vi "Set_2G_RACH_Transmission_Slots.vi"(8 "error in (no error)":errorcluster, 10 "value":i32=14 min=1 max=16, 11 "Base Station":T1) -> (0 "error out":errorcluster, 3 "Output String":string)   [LabVIEW 2021]
uses:
  Controls/Base_Station_Emulator.ctl
  Controls/TCP_FGV.ctl
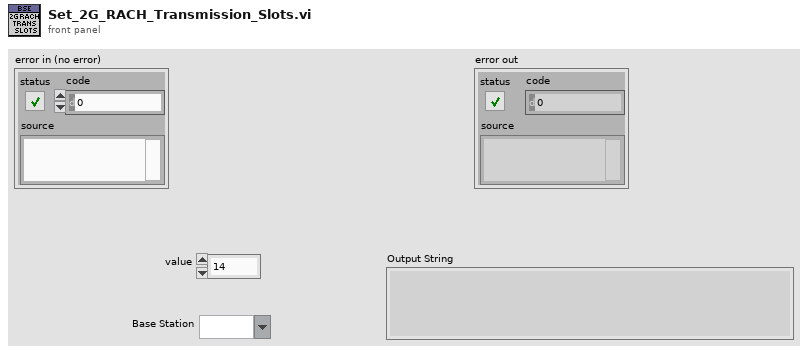
[diagram p1: front panel]
types:
  T1 = typedef "Base_Station_Emulator.ctl" = string
  T2 = typedef "TCP_FGV.ctl" = enum16{"Open", "Read", "Write", "Close"}
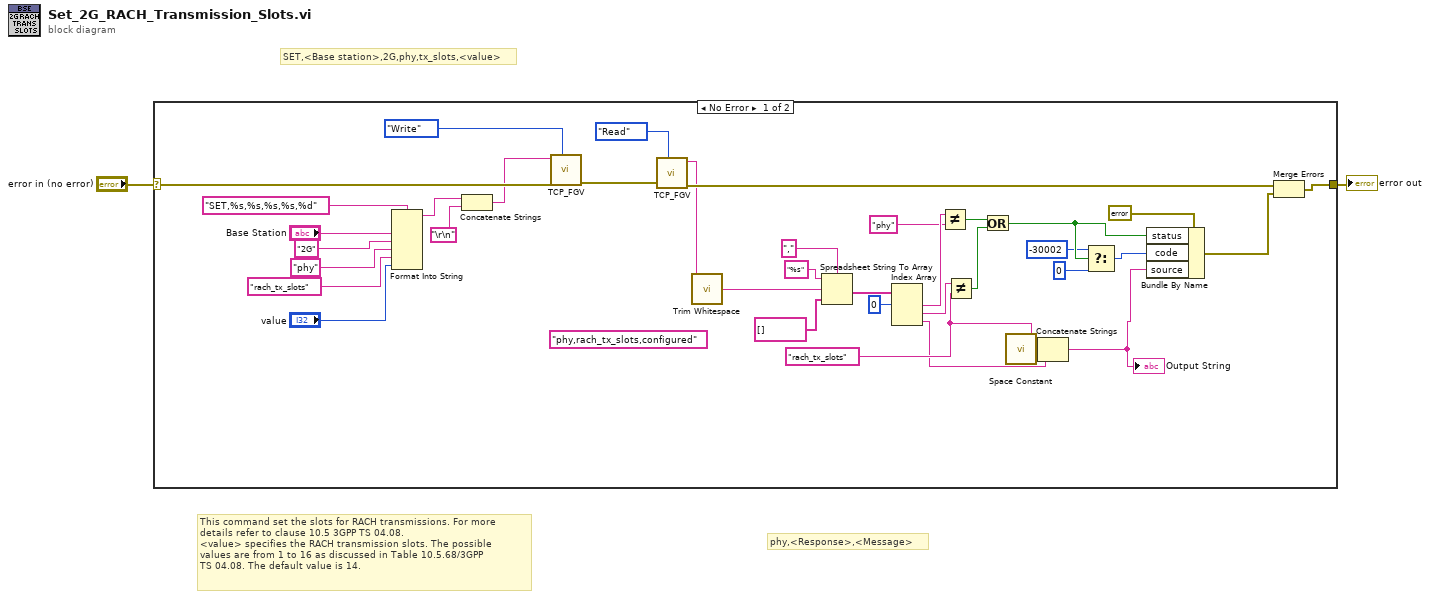
[diagram p0: block diagram]
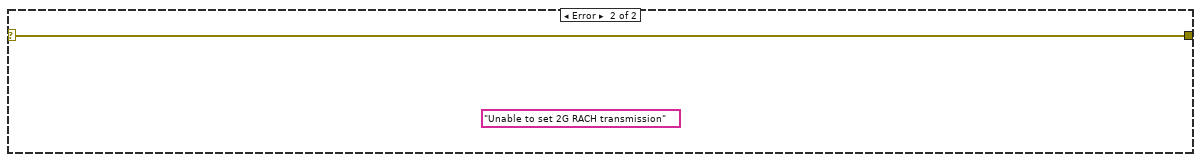
[diagram p2: hidden frame]
diagram:
  # "This command set the slots for RACH transmissions. For more \ndetails refer to clause 10.5 3GPP TS 04.08. \n<value> specifies the RACH transmission slots. The possible \nvalues are from 1 to 16 as discussed in Table 10.5.68/3GPP \nTS 04.08. The default value is 14."
  # "phy,<Response>,<Message>"
  # "SET,<Base station>,2G,phy,tx_slots,<value>"
  n1 = case shown="No Error" "error in (no error)" {
    selector: "error in (no error)" -> [w36 w40]
    tunnel: [w12 w40] -> w1
    frame No Error {
      (unwired) "phy,rach_tx_slots,configured" ("format string")
      w10 = "rach_tx_slots"
      n2 = Format Into String(format string="SET,%s,%s,%s,%s,%d", "Base Station", "2G", "phy", "rach_tx_slots", "value") -> (resulting string=w4:string)  [unwired: 2 in, 1 out]
      n3 = Concatenate Strings(w4, "\r\n") -> (w3:string)
      n4 = call "TCP_FGV.vi"("Command"=w3, "error in (no error)"=w36, "Operation"=TCP_FGV."Write") -> ("error out"=w13:errorcluster)  [unwired: 6 in, 1 out]
      n5 = call "TCP_FGV.vi"("error in (no error)"=w13, "Operation"=TCP_FGV."Read") -> ("Data Out"=w14:string, "error out"=w16:errorcluster)  [unwired: 7 in]
      n6 = call <vilib>:"Trim Whitespace.vi"("string"=w14) -> ("trimmed string"=w30:string)  [unwired: 1 in]
      n7 = Spreadsheet String To Array(delimiter (Tab)=",", format string="%s", spreadsheet string=w30, array type (2D Dbl)=string[] []) -> (array=w26:string[])
      n8 = Index Array(array=w26, index #1=0 ("index")) -> (element #1=w27:string, element #2=w17:string, element #3=w9:string)  [unwired: 2 in]
      n9 = Not Equal?(x=w27, y="phy" ("format string")) -> (x != y?=w28:bool)
      n10 = Not Equal?(x=w17, y=w10) -> (x != y?=w29:bool)
      n11 = Or(x=w28, y=w29) -> (x .or. y?=w31:bool)
      n12 = call <vilib>:"Space Constant.vi"() -> ("String"=w11:string)
      n13 = Concatenate Strings(w10, w11, w9) -> (w8:string)
      "Output String" <- w8
      n14 = Select(t=-30002 ("code"), s=w31, f=0 ("code")) -> (s? t:f=w32:i32)
      n15 = Bundle By Name(cluster=errorcluster {"status"=FALSE, "code"=0, "source"=""} ("error constant"), "status"=w31, "code"=w32, "source"=w8) -> (w15:errorcluster)
      n16 = Merge Errors(w16, w15) -> (w12:errorcluster)
    }
    frame Error {
      (unwired) "Unable to set 2G RACH transmission" ("source")
    }
  }
  "error out" <- w1
